vi "replace non-alphanumeric characters in string.vi"(9 "replace with (_)":string="_", 11 "string in":string) -> (3 "string out":string)   [LabVIEW 2014, in "Shared Memory editor node.lvclass"]
uses:
  Shared Memory editor node.lvclass
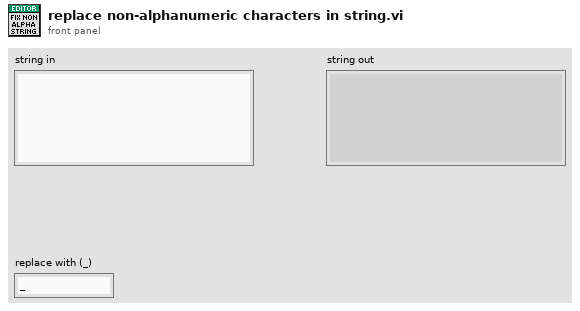
[diagram p1: front panel]
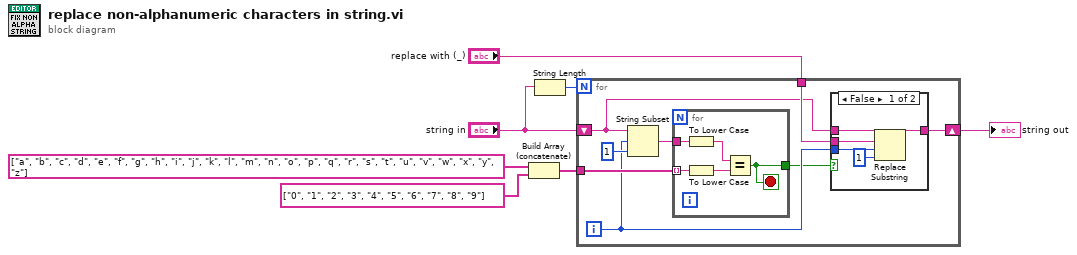
[diagram p0: block diagram]
diagram:
  n1 = Build Array (concatenate)(string[] ["a", "b", "c", "d", "e", "f", "g", "h", "i", "j", "k", "l", "m", "n", "o", "p", "q", "r", "s", "t", "u", "v", "w", "x", "y", "z"], string[] ["0", "1", "2", "3", "4", "5", "6", "7", "8", "9"]) -> (w4:string[])
  n2 = String Length(string="string in") -> (length=w6:i32)
  n3 = for {
    N: w6 -> [_]
    tunnel: w4 -> [w13]
    tunnel: "replace with (_)" -> [w9]
    shift-right: [w10] -> w3
    shift-left: "string in" -> [w8]
    i -> [w12]
    n4 = String Subset(string=w8, offset (0)=w12, length (rest)=1 ("length (rest)")) -> (substring=w14:string)
    n5 = for {
      tunnel: w14 -> [w24]
      tunnel: w13 -> [w26] mode=indexing
      tunnel: [w25] -> w11
      stop <- w25 stop-if-true
      n6 = To Lower Case(string=w24) -> (all lower case string=w23:string)
      n7 = To Lower Case(string=w26) -> (all lower case string=w22:string)
      n8 = Equal?(x=w23, y=w22) -> (x = y?=w25:bool)
    }
    n9 = case shown="False" w11 {
      tunnel: w12 -> [w20 _]
      tunnel: w8 -> [w19 w21]
      tunnel: w9 -> [w18 _]
      tunnel: [w17 w21] -> w10
      frame False {
        n10 = Replace Substring(2:1 ("length (len. of substring)"), 3:w20, 4:w18, 5:w19) -> (1:w17:string)  [unwired: 1 out]
      }
      frame True {
      }
    }
  }
  "string out" <- w3
